vi "Basic Control Panel.vi"() -> ()   [LabVIEW 2012]
doc: "This VI form sets all the set points for the current memory location.\nDESCRIPTION:\nThis VI configures the power supplies to generate a DV voltage at the output.\n\nINSTRUCTIONS:\n1. Enter the resource name.\n2. Enter voltage level, current limit, OVP limit and OCP limit.\n3. Set output enabled switch to ON if you want the generated voltage to appear at the instrument's output.\n4. Run the VI."
uses:
  Global/GPIB Numbers.vi
panel:
  in  "Set Current and Voltage":bool
  in  "stop":bool
  in  "Power":bool
  in  "error in (no error)":errorcluster
  out "Current":string
  out "Voltage":string
  in  "OCP":dbl format="%.2f"
  in  "OVP":dbl format="%.2f"
  in  "Current":dbl format="%.2f"
  in  "Voltage":dbl format="%.2f"
  # "MAGNA-POWER"
  # "Electronics"
  # "ON"
  # "OFF"
  # "Instrument Settings"
  # "Output Values"
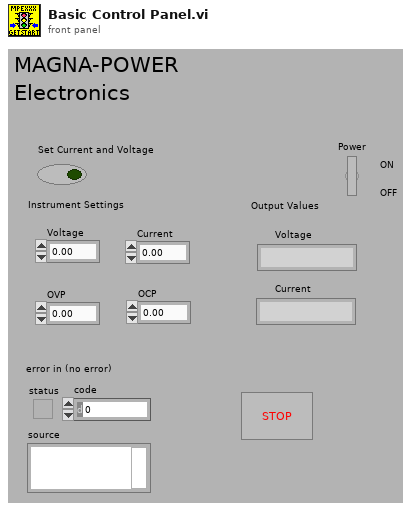
[diagram p1: front panel]
types:
  T1 = cluster{"Name":string, "bus":dbl, "GPIB":dbl, "GPIB as string":string, "byte":i32, "IVI resource name":refnum<k15>, "VISA Resource Name":refnum<visa-resource-name>}
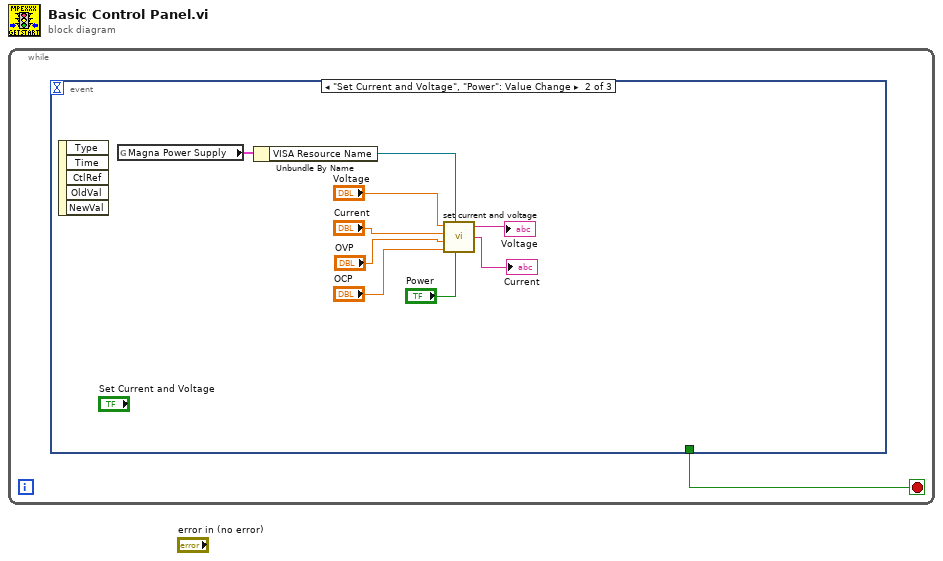
[diagram p0: block diagram]
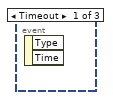
[diagram p2: hidden frame]
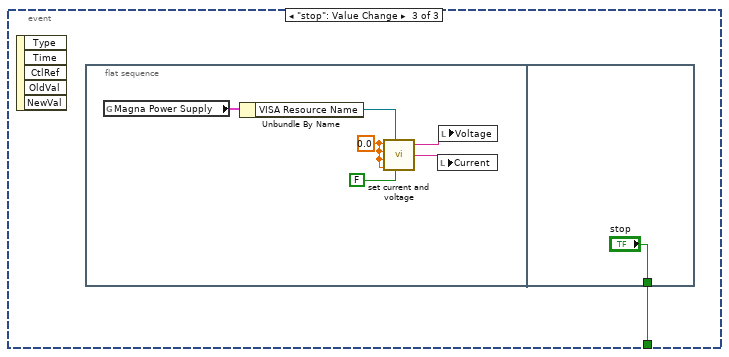
[diagram p3: hidden frame]
diagram:
  n1 = while {
    stop <- w1 stop-if-true
    n2 = event shown="[1] \"Set Current and Voltage\", \"Power\": Value Change" {
      selector: _ -> [_ _ _]
      dyn-events: _ -> [_ _ _]
      timeout: _ -> [_ _ _]
      tunnel: [_ _ w11] -> w1
      event Timeout {
        n3 = event-data() -> ()  [unwired: 1 in, 2 out]
      }
      event "Set Current and Voltage", "Power": Value Change {
        n4 = event-data() -> ()  [unwired: 1 in, 5 out]
        n5 = global read "GPIB Numbers.vi" "Magna Power Supply"() -> (w9:T1)
        n6 = Unbundle By Name(w9) -> ("VISA Resource Name"=w8:refnum<visa-resource-name>)
        n7 = call "set current and voltage.vi"("Voltage"="Voltage", "VISA Resource Name"=w8, "Current"="Current", "OVP"="OVP", "Power"="Power", "OCP"="OCP") -> ("Voltage"=→"Voltage":string, "Current"=→"Current":string)  [unwired: 1 in]
      }
      event "stop": Value Change {
        n8 = event-data() -> ()  [unwired: 1 in, 5 out]
        n9 = flat-sequence {
          tunnel: ["stop"] -> w11
          frame #0 {
            w15 = 0.0 ("Voltage")
            n10 = global read "GPIB Numbers.vi" "Magna Power Supply"() -> (w17:T1)
            n11 = Unbundle By Name(w17) -> ("VISA Resource Name"=w16:refnum<visa-resource-name>)
            n12 = call "set current and voltage.vi"("Voltage"=w15, "VISA Resource Name"=w16, "Current"=w15, "OVP"=w15, "Power"=FALSE, "OCP"=w15) -> ("Voltage"=w12:string, "Current"=w13:string)  [unwired: 1 in]
            n13 = local write "Current"(w13) -> ()
            n14 = local write "Voltage"(w12) -> ()
          }
          frame #1 {
          }
        }
      }
    }
  }
